vi "CreatePrivateEvents.vi"(8 "error in (no error)":errorcluster, 11 "LockinDAQ":refnum<class "LockinDAQ.lvclass">) -> (0 "error out":errorcluster, 3 "LockinDAQ out":refnum<class "LockinDAQ.lvclass">)   [LabVIEW 2016, in "LockinDAQ.lvclass"]
doc: "---------------------------------------------------------------\nJKI State Machine Objects™\nhttp://jki.net/state-machine-objects/\nCopyright (C) 2005-2015, JKI <info@jki.net>\nALL RIGHTS RESERVEDJKI State Machine Objects (SMO) 1.0.0.4\nJKI - JKI\nCopyright (c) 2015, JKI"
uses:
  LockinDAQ.lvclass
  Typedefs/PrivateEvents--LockinDAQ.setAOconfig.ctl
  Typedefs/AO.config-array.ctl
  Typedefs/AO.config-cluster.ctl
  Typedefs/446xAO-enum.ctl
  Typedefs/DAQType-enum.ctl
  Typedefs/PrivateEvents--LockinDAQ.setAIconfig.ctl
  Typedefs/AI.config-array.ctl
  Typedefs/AI.config-cluster.ctl
  Typedefs/AI.coupling-enum.ctl
  Typedefs/446xAI-enum.ctl
  Typedefs/AI Simulation-enum.ctl
  Typedefs/PrivateEvents--LockinDAQ.setAO.ctl
  Typedefs/AO-cluster.ctl
  Typedefs/Function-enum.ctl
  Typedefs/PrivateEvents--LockinDAQ.setREF.ctl
  Typedefs/REF-cluster.ctl
  Typedefs/PrivateEvents--LockinDAQ.setSampling.ctl
  Typedefs/Sampling.ctl
  Typedefs/Sample Mode--Ring.ctl
  Typedefs/PrivateEvents--LockinDAQ.setState.ctl
  Typedefs/Set State-enum.ctl
  Typedefs/PrivateEvents--LockinDAQ.setGain.ctl
  Typedefs/PrivateEvents--LockinDAQ.setSweep.ctl
  Typedefs/Sweep Configuration--Cluster.ctl
  Typedefs/PrivateEvents--LockinDAQ.measureOffset.ctl
  Typedefs/PrivateEvents--LockinDAQ.zeroOffset.ctl
  Typedefs/PrivateEvents--LockinDAQ.setPreFilter.ctl
  Typedefs/AI Prefilter-cluster.ctl
  Typedefs/PrivateEvents--LockinDAQ.autoContigureDAQ.ctl
  LockinDAQ.lvclass/LockinDAQ.ctl
  <userlib>/LevyLab/Levylab Instruments/SMOs/LevyLab/LevyLab.lvclass
panel:
  # "For instructions on how to use the JKI State Machine Objects, examples and video tutorials, visit:\nhttp://jki.net/state-machine-objects/\n\nJKI State Machine Objects™\nhttp://jki.net/state-machine-objects/\nCopyright (C) 2005-2015, JKI <info@jki.net>\nALL RIGHTS RESERVED"
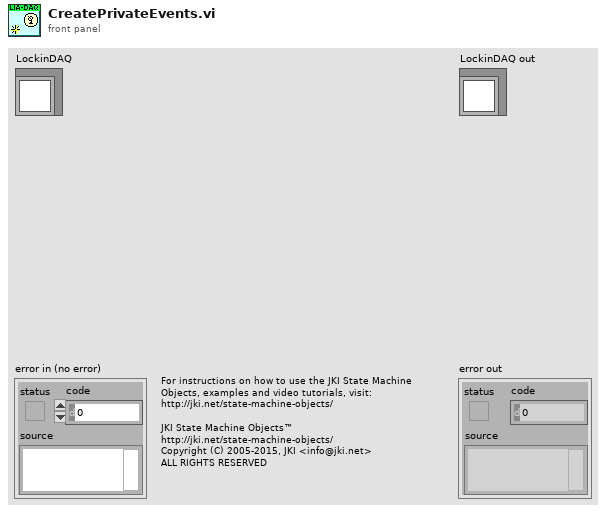
[diagram p1: front panel]
types:
  T1 = typedef "LockinDAQ.lvclass/PrivateEvents--LockinDAQ.autoContigureDAQ.ctl" = bool
  T2 = typedef "LockinDAQ.lvclass/PrivateEvents--LockinDAQ.setPreFilter.ctl" = cluster{"PreFilter":T3}
  T3 = typedef "LockinDAQ.lvclass/AI Prefilter-cluster.ctl" = cluster{"60 Hz prefilter":bool, "LP prefilter":bool, "LP cutoff (Hz)":dbl}
  T4 = typedef "LockinDAQ.lvclass/PrivateEvents--LockinDAQ.zeroOffset.ctl" = bool
  T5 = typedef "LockinDAQ.lvclass/PrivateEvents--LockinDAQ.measureOffset.ctl" = bool
  T6 = typedef "LockinDAQ.lvclass/PrivateEvents--LockinDAQ.setSweep.ctl" = cluster{"setSweep":T7}
  T7 = typedef "LockinDAQ.lvclass/Sweep Configuration--Cluster.ctl" = cluster{"Sweep Type":enum16{"sweepLockin", "sweepIV"}, "Sweep Lockin Time (s)":dbl, "Sweep IV Step (V)":dbl, "Initial Wait Time (s)":dbl, "Sweep Channel":i32[], "Sweep Start (V)":dbl[], "Sweep End (V)":dbl[], "Return to Start":bool}
  T8 = typedef "LockinDAQ.lvclass/PrivateEvents--LockinDAQ.setGain.ctl" = dbl[]
  T9 = typedef "LockinDAQ.lvclass/PrivateEvents--LockinDAQ.setState.ctl" = cluster{"setState":T10}
  T10 = typedef "LockinDAQ.lvclass/Set State-enum.ctl" = enum16{"start", "stop", "reset", "calibrate", "start sweep", "stop sweep"}
  T11 = typedef "LockinDAQ.lvclass/PrivateEvents--LockinDAQ.setSampling.ctl" = cluster{"Sampling":T12, "Sample Mode":T13, "AI Buffer Size (S)":i32, "Decimation":i32}
  T12 = typedef "LockinDAQ.lvclass/Sampling.ctl" = cluster{"Fs":dbl, "#s":i32}
  T13 = typedef "LockinDAQ.lvclass/Sample Mode--Ring.ctl" = i32
  T14 = typedef "LockinDAQ.lvclass/PrivateEvents--LockinDAQ.setREF.ctl" = cluster{"Channels: Lockin":T15}
  T15 = typedef "LockinDAQ.lvclass/REF-cluster.ctl" = cluster{"Ch":i32[], " f (Hz)":dbl[], "Phase (°)":dbl[], "TC (s)":dbl[], "order":i32[]}
  T16 = typedef "LockinDAQ.lvclass/PrivateEvents--LockinDAQ.setAO.ctl" = cluster{"Channels: AO":T17}
  T17 = typedef "LockinDAQ.lvclass/AO-cluster.ctl" = cluster{"Ch":i32[], "Amp (V)":dbl[], "DC (V)":dbl[], "f (Hz)":dbl[], "Phase (°)":dbl[], "Function":T18[], "Sweep?":bool[]}
  T18 = typedef "LockinDAQ.lvclass/Function-enum.ctl" = enum16{"Sine", "Triangle", "Square", "Sawtooth"}
  T19 = typedef "LockinDAQ.lvclass/PrivateEvents--LockinDAQ.setAIconfig.ctl" = cluster{"AI Configuration":T20, "Simulation mode":T25}
  T20 = typedef "LockinDAQ.lvclass/AI.config-array.ctl" = T21[]
  T21 = typedef "LockinDAQ.lvclass/AI.config-cluster.ctl" = cluster{"AI.channels":tag, "AI.Coupling":T22, "AI.Range":T23, "input terminal configuration":i32, "DAQ Type":T24}
  T22 = typedef "LockinDAQ.lvclass/AI.coupling-enum.ctl" = u16
  T23 = typedef "LockinDAQ.lvclass/446xAI-enum.ctl" = enum16{"±0.316 V", "±1.00 V", "±3.16 V", "±10.0 V", "±31.6 V", "±42.4 V"}
  T24 = typedef "LockinDAQ.lvclass/DAQType-enum.ctl" = enum16{"None", "USB 4431", "PXI 446x"}
  T25 = typedef "LockinDAQ.lvclass/AI Simulation-enum.ctl" = enum16{"AI = HW simulated", "AI = noise*AO", "AI = waveguide"}
  T26 = typedef "LockinDAQ.lvclass/PrivateEvents--LockinDAQ.setAOconfig.ctl" = cluster{"AO Configuration":T27}
  T27 = typedef "LockinDAQ.lvclass/AO.config-array.ctl" = T28[]
  T28 = typedef "LockinDAQ.lvclass/AO.config-cluster.ctl" = cluster{"AO.channels":tag, "AO.Range":T29, "output terminal configuration":i32, "DAQ Type":T24}
  T29 = typedef "LockinDAQ.lvclass/446xAO-enum.ctl" = enum16{"±0.1 V", "±1.0 V", "±10.0 V"}
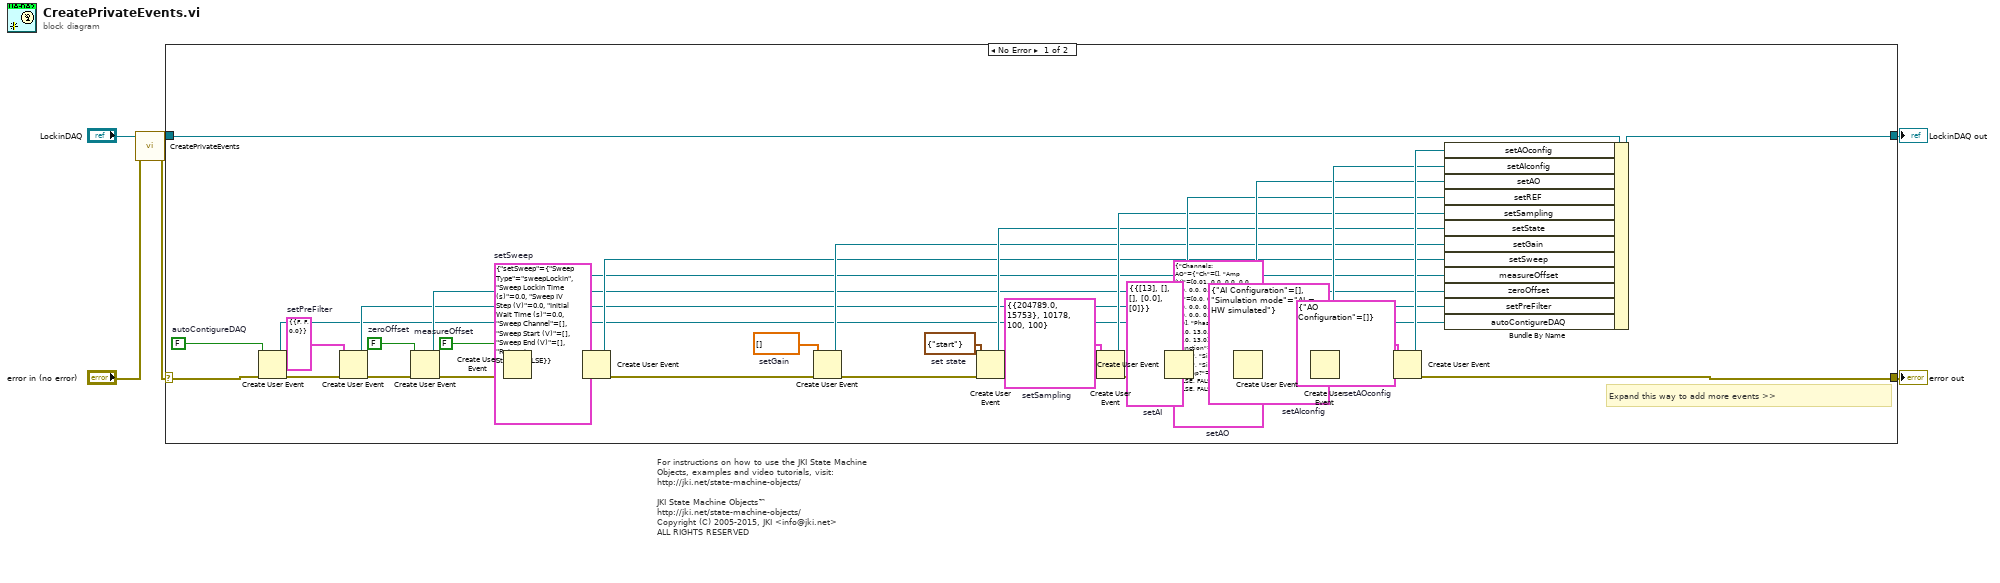
[diagram p0: block diagram]
diagram:
  # "For instructions on how to use the JKI State Machine Objects, examples and video tutorials, visit:\nhttp://jki.net/state-machine-objects/\n\nJKI State Machine Objects™\nhttp://jki.net/state-machine-objects/\nCopyright (C) 2005-2015, JKI <info@jki.net>\nALL RIGHTS RESERVED"
  n1 = call-parent "CreatePrivateEvents.vi"("error in (no error)"="error in (no error)", "SMO"="LockinDAQ") -> ("error out"=w1:errorcluster, "SMO out"=w3:refnum<class "LockinDAQ.lvclass">)  [unwired: 8 in]
  n2 = case shown="No Error" w1 {
    selector: w1 -> [w44 w47]
    tunnel: [w42 w47] -> w5
    tunnel: [w43 w46] -> w6
    tunnel: w3 -> [w45 w46]
    frame No Error {
      w8 = T1 FALSE  # autoContigureDAQ
      w11 = T2 {"PreFilter"={"60 Hz prefilter"=FALSE, "LP prefilter"=FALSE, "LP cutoff (Hz)"=0.0}}  # setPreFilter
      w14 = T4 FALSE  # zeroOffset
      w17 = T5 FALSE  # measureOffset
      w20 = T6 {"setSweep"={"Sweep Type"=enum."sweepLockin", "Sweep Lockin Time (s)"=0.0, "Sweep IV Step (V)"=0.0, "Initial Wait Time (s)"=0.0, "Sweep Channel"=[], "Sweep Start (V)"=[], "Sweep End (V)"=[], "Return to Start"=FALSE}}  # setSweep
      w23 = T8 []  # setGain
      w26 = T9 {"setState"=enum."start"}  # set state
      w29 = T11 {"Sampling"={"Fs"=204789.0, "#s"=15753}, "Sample Mode"=10178, "AI Buffer Size (S)"=100, "Decimation"=100}  # setSampling
      w32 = T14 {"Channels: Lockin"={"Ch"=[13], " f (Hz)"=[], "Phase (°)"=[], "TC (s)"=[0.0], "order"=[0]}}  # setAI
      w35 = T16 {"Channels: AO"={"Ch"=[], "Amp (V)"=[0.01, 0.0, 0.0, 0.0, 0.0, 0.0, 0.0, 0.0], "DC (V)"=[0.0, 0.0, 0.0, 0.0, 0.0, 0.0, 0.0, 0.0], "f (Hz)"=[0.0, 0.0, 0.0, 0.0, 0.0, 0.0, 0.0, 0.0], "Phase (°)"=[13.1, 13.0, 13.0, 13.0, 13.0, 13.0, 13.0, 13.0], "Function"=[enum."Sine", enum."Sine", enum."Sine", enum."Sine", enum."Sine", enum."Sine", enum."Sine", enum."Sine"], "Sweep?"=[FALSE, FALSE, FALSE, FALSE, FALSE, FALSE, FALSE, FALSE]}}  # setAO
      w38 = T19 {"AI Configuration"=[], "Simulation mode"=enum."AI = HW simulated"}  # setAIconfig
      w41 = T26 {"AO Configuration"=[]}  # setAOconfig
      # "Expand this way to add more events >>"
      n3 = Create User Event(user event datatype=w8, error in=w44) -> (user event=w7:refnum<user-event>, error out=w9:errorcluster)
      n4 = Create User Event(user event datatype=w11, error in=w9) -> (user event=w10:refnum<user-event>, error out=w12:errorcluster)
      n5 = Create User Event(user event datatype=w14, error in=w12) -> (user event=w13:refnum<user-event>, error out=w15:errorcluster)
      n6 = Create User Event(user event datatype=w17, error in=w15) -> (user event=w16:refnum<user-event>, error out=w18:errorcluster)
      n7 = Create User Event(user event datatype=w20, error in=w18) -> (user event=w19:refnum<user-event>, error out=w21:errorcluster)
      n8 = Create User Event(user event datatype=w23, error in=w21) -> (user event=w22:refnum<user-event>, error out=w24:errorcluster)
      n9 = Create User Event(user event datatype=w26, error in=w24) -> (user event=w25:refnum<user-event>, error out=w27:errorcluster)
      n10 = Create User Event(user event datatype=w29, error in=w27) -> (user event=w28:refnum<user-event>, error out=w30:errorcluster)
      n11 = Create User Event(user event datatype=w32, error in=w30) -> (user event=w31:refnum<user-event>, error out=w33:errorcluster)
      n12 = Create User Event(user event datatype=w35, error in=w33) -> (user event=w34:refnum<user-event>, error out=w36:errorcluster)
      n13 = Create User Event(user event datatype=w38, error in=w36) -> (user event=w37:refnum<user-event>, error out=w39:errorcluster)
      n14 = Create User Event(user event datatype=w41, error in=w39) -> (user event=w40:refnum<user-event>, error out=w42:errorcluster)
      n15 = Bundle By Name(cluster=w45, "setAOconfig"=w40, "setAIconfig"=w37, "setAO"=w34, "setREF"=w31, "setSampling"=w28, "setState"=w25, "setGain"=w22, "setSweep"=w19, "measureOffset"=w16, "zeroOffset"=w13, "setPreFilter"=w10, "autoContigureDAQ"=w7) -> (w43:refnum<class "LockinDAQ.lvclass">)
    }
    frame Error {
    }
  }
  "error out" <- w5
  "LockinDAQ out" <- w6
